vi "Close.vi"(8 "error in (no error)":errorcluster, 11 "Ismatech 3 Channel Settings In":T1={"VISA resource name"="", "Pump Number"=1, "Channel Number"=0, "Simulated?"=TRUE, "Reverse?"=FALSE} {"Channel Number" min=0 max=3; "Pump Number" min=1 max=9}) -> (0 "error out":errorcluster, 1 "Connection Error":bool, 3 "Ismatech 3 Channel Settings Out":T1={"VISA resource name"="", "Pump Number"=1, "Channel Number"=0, "Simulated?"=TRUE, "Reverse?"=FALSE} {"Channel Number" min=0 max=3; "Pump Number" min=1 max=9})   [LabVIEW 2018, in "Ismatec 4308.lvlib"]
uses:
  Ismatec 4308.lvlib
  Ismatec 4083.ctl
  support/Support Library.lvlib
panel:
  out "read buffer":string
  out "Failed to stop":bool
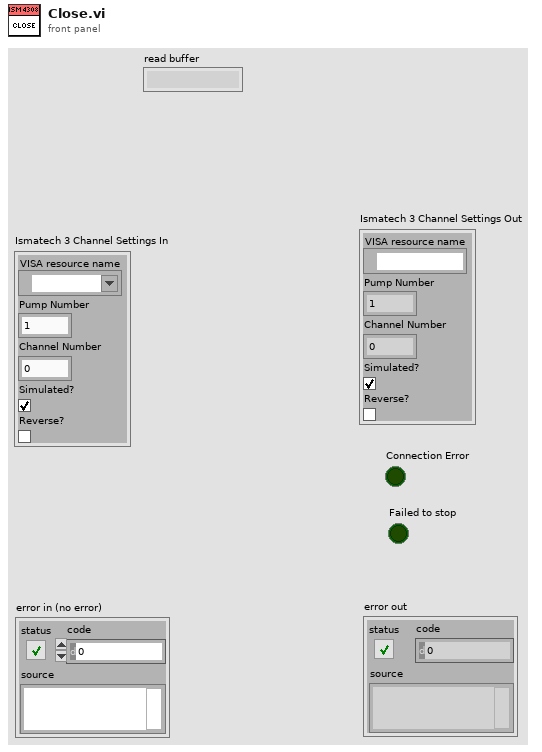
[diagram p1: front panel]
types:
  T1 = typedef "Ismatec 4308.lvlib/Ismatec 4083.ctl" = cluster{"VISA resource name":refnum<visa-resource-name>, "Pump Number":i16, "Channel Number":i16, "Simulated?":bool, "Reverse?":bool}
  T2 = typedef "Ismatec 4308.lvlib/Ismatec 4083 Global.ctl" = T3[]
  T3 = typedef "Ismatec 4308.lvlib/Ismatec 4083 Global Element.ctl" = cluster{"Busy":bool, "ChannelCnt":dbl, "Initialized":bool, "Current Channel":dbl, "Initialized Channels":dbl[]}
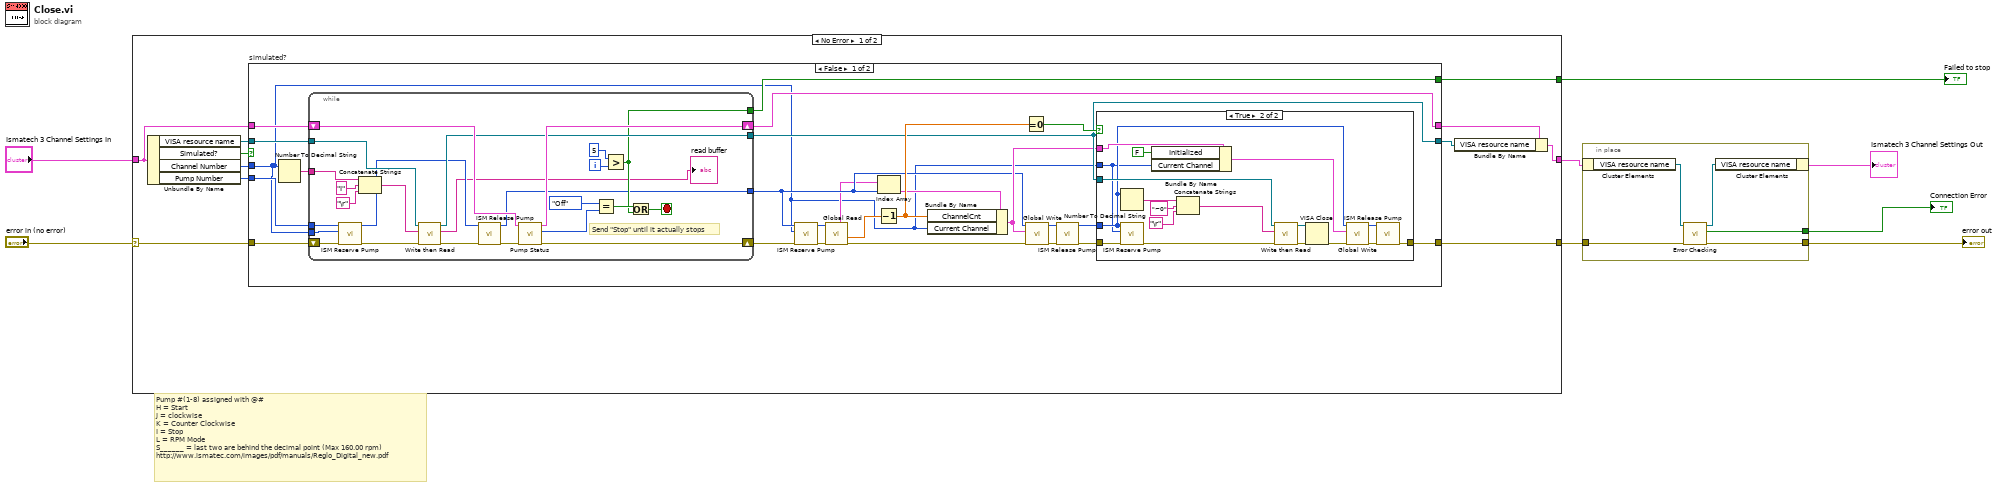
[diagram p0: block diagram]
diagram:
  # "Pump #(1-8) assigned with @#\nH = Start\nJ = clockwise\nK = Counter Clockwise\nI = Stop\nL = RPM Mode\nS______ = last two are behind the decimal point (Max 160.00 rpm)\nhttp://www.ismatec.com/images/pdf/manuals/Reglo_Digital_new.pdf"
  n1 = case shown="No Error" "error in (no error)" {
    selector: "error in (no error)" -> [w14 w93]
    tunnel: [w18 w93] -> w7
    tunnel: [w15 w92] -> w4
    tunnel: "Ismatech 3 Channel Settings In" -> [w11 w92]
    tunnel: [w9 _] -> w1
    frame No Error {
      n2 = Unbundle By Name(w11) -> ("VISA resource name"=w13:refnum<visa-resource-name>, "Simulated?"=w19:bool, "Channel Number"=w16:i16, "Pump Number"=w10:i16)
      n3 = case "simulated?" shown="False" w19 {
        tunnel: [w33 w89] -> w18
        tunnel: [w34 w90] -> w17
        tunnel: w16 -> [w20 _]
        tunnel: w14 -> [w44 w89]
        tunnel: w13 -> [w43 w90]
        tunnel: w11 -> [w42 w91]
        tunnel: [w41 w91] -> w12
        tunnel: w10 -> [w25 _]
        tunnel: [w39 _] -> w9
        frame False {
          n4 = Number To Decimal String(number=w20) -> (decimal integer string=w40:string)  [unwired: 1 in]
          n5 = while {
            tunnel: w43 -> [w86]
            shift-right: [w87] -> w32
            shift-left: w44 -> [w79]
            shift-right: [w84] -> w41
            shift-left: w42 -> [w85]
            tunnel: [w82] -> w34
            tunnel: w40 -> [w80]
            tunnel: w25 -> [w78]
            tunnel: [w71] -> w39
            tunnel: [w65] -> w22
            tunnel: w20 -> [w64]
            i -> [w75]
            stop <- w72 stop-if-true
            # "Send \"Stop\" until it actually stops"
            n6 = call "ISM Reserve Pump.vi"("error in (no error)"=w79, "ISM Channel # In"=w64, "ISM Pump # In"=w78) -> ("error out"=w77:errorcluster, "ISM Pump # Out"=w76:i32)  [unwired: 7 in]
            n7 = Concatenate Strings(w80, "I" ("string"), "\r") -> (w68:string)
            n8 = call "Write then Read.vi"("error in"=w77, "write buffer"=w68, "VISA resource name in"=w86) -> ("error out"=w67:errorcluster, "read buffer"=→"read buffer":string, "VISA resource name out"=w82:refnum<visa-resource-name>)  [unwired: 6 in]
            n9 = call "ISM Release Pump.vi"("error in (no error)"=w67, "Pump Number In"=w76) -> ("error out"=w88:errorcluster, "Pump Number Out"=w65:i32)  [unwired: 8 in]
            n10 = call "Pump Status.vi"("error in (no error)"=w88, "Ismatech 3 Channel Settings In"=w85) -> ("error out"=w87:errorcluster, "Pump On?"=w83:enum16{"Off", "On", "Not Initialized"}, "Ismatech 3 Channel Settings Out"=w84:T1)  [unwired: 5 in, 2 out]
            n11 = Equal?(x=enum16{"Off", "On", "Not Initialized"}."Off", y=w83) -> (x = y?=w73:bool)
            n12 = Greater?(x=5, y=w75) -> (0:w71:bool)
            n13 = Or(x=w73, y=w71) -> (x .or. y?=w72:bool)
          }
          n14 = call "ISM Reserve Pump.vi"("error in (no error)"=w32, "ISM Channel # In"=w20, "ISM Pump # In"=w22) -> ("error out"=w30:errorcluster, "ISM Pump # Out"=w31:i32)  [unwired: 7 in]
          n15 = call "Global Read.vi"("error in (no error)"=w30, "Pump Number"=w31) -> ("error out"=w37:errorcluster, "ChannelCnt"=w38:dbl, "Ismatec 4083 Global"=w21:T2)  [unwired: 3 in, 4 out]
          n16 = Index Array(array=w21, index=w22) -> (element=w24:T3)
          n17 = Decrement(x=w38) -> (x-1=w35:dbl)
          n18 = Bundle By Name(cluster=w24, "ChannelCnt"=w35, "Current Channel"=w20) -> (w23:T3)
          n19 = Equal To 0?(x=w35) -> (x = 0?=w36:bool)
          n20 = call "Global Write.vi"("error in (no error)"=w37, "Incoming Cluster"=w23, "Pump Number In"=w22) -> ("error out"=w28:errorcluster, "Pump Number Out"=w29:i32)  [unwired: 7 in]
          n21 = call "ISM Release Pump.vi"("error in (no error)"=w28, "Pump Number In"=w29) -> ("error out"=w27:errorcluster, "Pump Number Out"=w26:i32)  [unwired: 8 in]
          n22 = case shown="True" w36 {
            tunnel: w26 -> [_ w48]
            tunnel: w34 -> [_ w53]
            tunnel: w27 -> [w45 w50]
            tunnel: [w45 w55] -> w33
            tunnel: w23 -> [_ w58]
            tunnel: w20 -> [_ w46]
            frame False {
            }
            frame True {
              n23 = Number To Decimal String(number=w48) -> (decimal integer string=w61:string)  [unwired: 1 in]
              n24 = call "ISM Reserve Pump.vi"("error in (no error)"=w50, "ISM Channel # In"=w46, "ISM Pump # In"=w48) -> ("error out"=w49:errorcluster)  [unwired: 7 in, 1 out]
              n25 = Bundle By Name(cluster=w58, "Initialized"=FALSE, "Current Channel"=w46) -> (w56:T3)
              n26 = Concatenate Strings(w61, "~0" ("string"), "\r") -> (w54:string)
              n27 = call "Write then Read.vi"("error in"=w49, "write buffer"=w54, "VISA resource name in"=w53) -> ("error out"=w51:errorcluster, "VISA resource name out"=w52:refnum<visa-resource-name>)  [unwired: 6 in, 1 out]
              n28 = VISA Close(VISA resource name=w52, error in (no error)=w51) -> (error out=w47:errorcluster)
              n29 = call "Global Write.vi"("error in (no error)"=w47, "Incoming Cluster"=w56, "Pump Number In"=w48) -> ("error out"=w60:errorcluster, "Pump Number Out"=w59:i32)  [unwired: 7 in]
              n30 = call "ISM Release Pump.vi"("error in (no error)"=w60, "Pump Number In"=w59) -> ("error out"=w55:errorcluster)  [unwired: 8 in, 1 out]
            }
          }
        }
        frame True {
        }
      }
      n31 = Bundle By Name(cluster=w12, "VISA resource name"=w17) -> (w15:T1)
    }
    frame Error {
    }
  }
  "Failed to stop" <- w1
  n32 = in-place {
    in-place-border: w7 -> [w98]
    in-place-border: [w97] -> w6
    in-place-border: [w96] -> w5
    n33 = in-place-cluster #1(w4) -> ("VISA resource name"=w95:refnum<visa-resource-name>)
    n34 = call "Error Checking.vi"("error in (no error)"=w98, "VISA resource name"=w95) -> ("error out"=w97:errorcluster, "Connection Error"=w96:bool, "VISA resource name"=w94:refnum<visa-resource-name>)  [unwired: 7 in]
    n35 = in-place-cluster #1("VISA resource name"=w94) -> (→"Ismatech 3 Channel Settings Out":T1)
  }
  "error out" <- w6
  "Connection Error" <- w5
